vi "laser_LED_controls.vi"(1 "Pulse Duty Cycle":dbl=50.0 caption="%" min=0.0 max=100.0 step=0.1, 2 "Pulse 488":bool, 3 "Zelux Frequency":u16=10 caption="Hz", 11 "Running":bool) -> ()   [LabVIEW 2025]
uses:
  channel parameters cluster.ctl
  <vilib>/Utility/error.llb/DialogType.ctl
  <vilib>/DAQmx/write.llb/DAQmx Write (Analog 1D DBL NChan 1Samp).vi
  <vilib>/DAQmx/miscellaneous.llb/DAQmx Fill In Error Info.vi
panel:
  in  "488 nm LED control":dbl(slide) step=1.0 scale=0.0..100.0 scale format="%#_3g"
  out "488  nm voltage":dbl
  out "594 nm voltage":dbl
  in  "594 nm laser control":dbl(slide) step=1.0 scale=0.0..100.0 scale format="%#_3g"
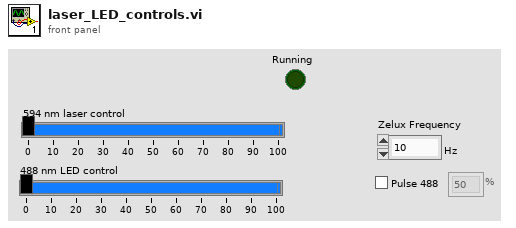
[diagram p1: front panel]
types:
  T1 = typedef "channel parameters cluster.ctl" = cluster{"voltage":dbl, "frequency":dbl, "duty cycle":dbl, "sample rate":dbl}
  T2 = typedef "DialogType.ctl" = u16
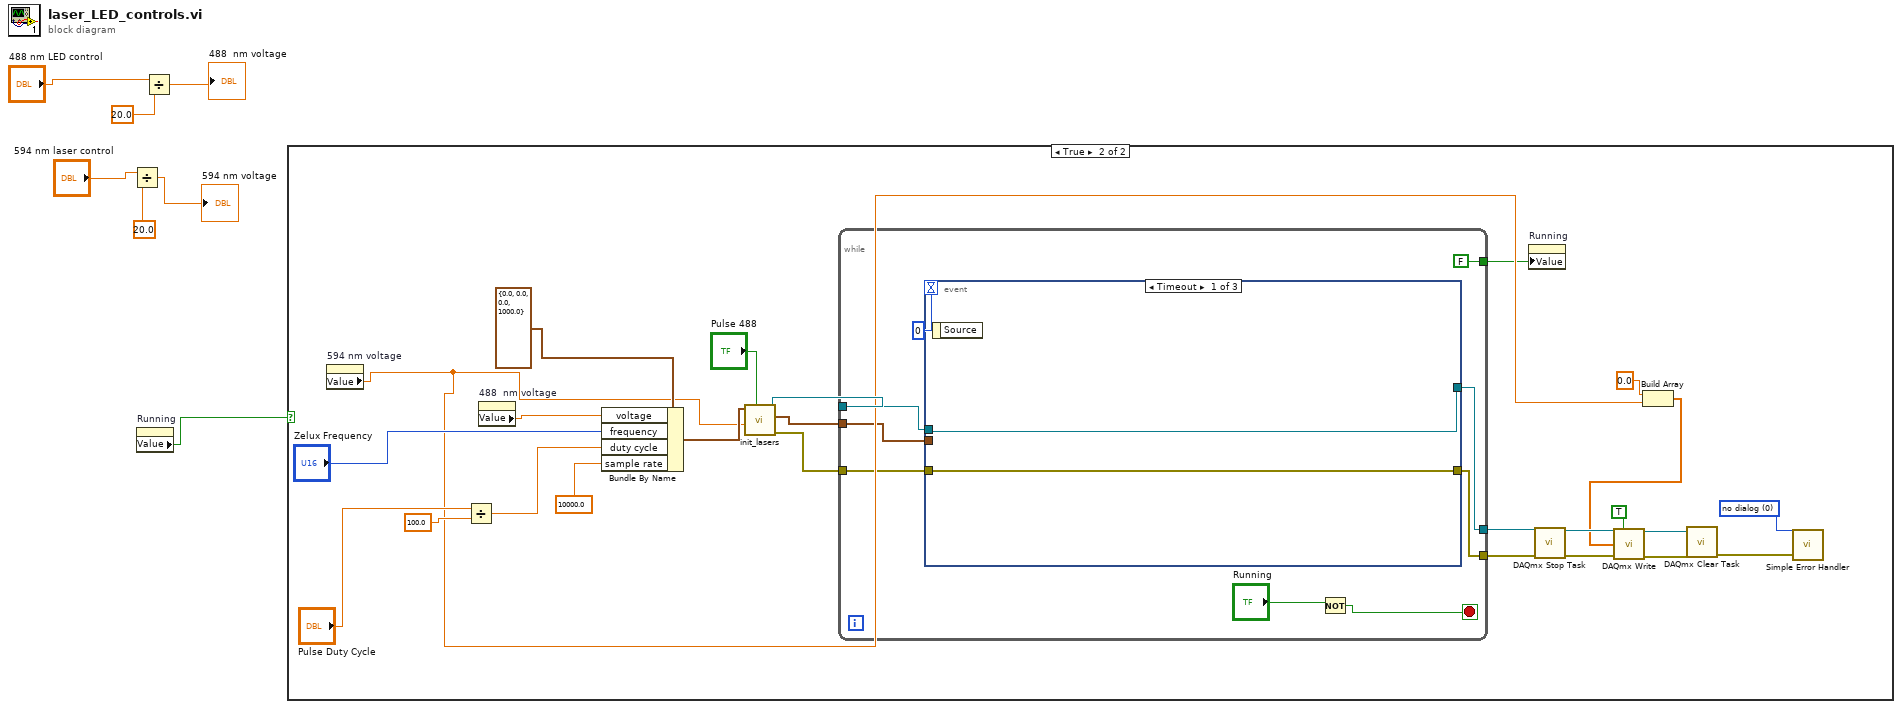
[diagram p0: block diagram]
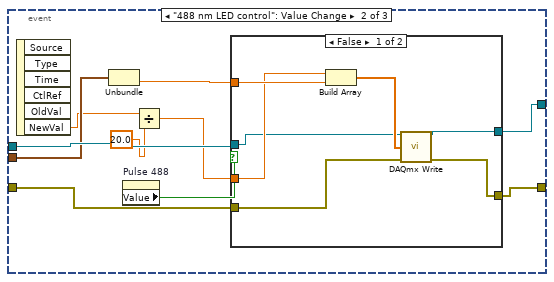
[diagram p3: hidden frame]
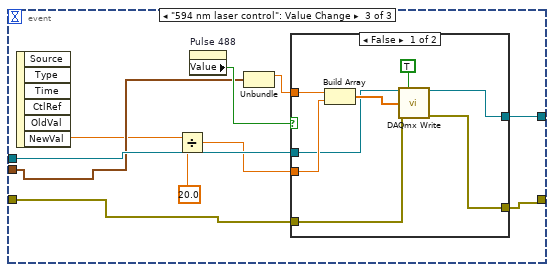
[diagram p5: hidden frame]
diagram:
  n1 = Divide(x="594 nm laser control", y=20.0) -> (x/y=→"594 nm voltage":dbl)
  n2 = property on="Running" class="Bool (strict)"() -> ("Value"=w1:bool)  [unwired: 2 in, 2 out]
  n3 = Divide(x="488 nm LED control", y=20.0) -> (x/y=→"488  nm voltage":dbl)
  n4 = case shown="True" w1 {
    frame False {
    }
    frame True {
      w22 = T2 0 items=["no dialog", "OK message", "continue or stop message", "OK message + warnings", "continue/stop + warnings"] ("type of dialog (OK msg:1)")
      n5 = property on="594 nm voltage" class="DigNum (strict)"() -> ("Value"=w13:dbl)  [unwired: 2 in, 2 out]
      n6 = Divide(x="Pulse Duty Cycle", y=100.0) -> (x/y=w30:dbl)
      n7 = property on="488  nm voltage" class="DigNum (strict)"() -> ("Value"=w27:dbl)  [unwired: 2 in, 2 out]
      n8 = Bundle By Name(cluster=T1 {"voltage"=0.0, "frequency"=0.0, "duty cycle"=0.0, "sample rate"=1000.0} ("channel parameters"), "voltage"=w27, "frequency"="Zelux Frequency", "duty cycle"=w30, "sample rate"=10000.0) -> (w32:T1)
      n9 = call "init_lasers.vi"("488 pulsed"="Pulse 488", "594 nm voltage"=w13, "488 nm channel parameters"=w32) -> ("error out"=w10:errorcluster, "current data"=w9:cluster{"[0]":dbl, "[1]":dbl}, "task out"=w15:refnum<k21>)  [unwired: 6 in]
      n10 = while {
        tunnel: w15 -> [w40]
        tunnel: w10 -> [w39]
        tunnel: [w38] -> w12
        tunnel: [w37] -> w11
        tunnel: w9 -> [w36]
        tunnel: [FALSE] -> w8
        stop <- w33 stop-if-true
        n11 = event shown="[0] Timeout" {
          selector: _ -> [_ _ _]
          dyn-events: _ -> [_ _ _]
          timeout: 0 -> [_ _ _]
          tunnel: w40 -> [w43 w51 w69]
          tunnel: w39 -> [w42 w52 w68]
          tunnel: [w43 w50 w70] -> w37
          tunnel: [w42 w47 w67] -> w38
          tunnel: w36 -> [_ w48 w66]
          event Timeout {
            n12 = event-data() -> ()  [unwired: 1 in, 1 out]
          }
          event "488 nm LED control": Value Change {
            n13 = event-data() -> ("NewVal"=w45:dbl)  [unwired: 1 in, 5 out]
            n14 = Unbundle(w48) -> ("[1]"=w49:dbl)  [unwired: 1 out]
            n15 = property on="Pulse 488" class="Bool (strict)"() -> ("Value"=w53:bool)  [unwired: 2 in, 2 out]
            n16 = Divide(x=w45, y=20.0) -> (x/y=w44:dbl)
            n17 = case shown="False" w53 {
              tunnel: [w59 w62] -> w47
              tunnel: w52 -> [w58 w62]
              tunnel: w51 -> [w54 w61]
              tunnel: [w57 w61] -> w50
              tunnel: w49 -> [w56 _]
              tunnel: w44 -> [w55 _]
              frame False {
                n18 = Build Array(w55, w56) -> (w60:dbl[])
                n19 = call-poly <vilib>:"DAQmx Write.vi"("task/channels in"=w54, "data"=w60, "error in"=w58) -> ("task out"=w57:refnum<k21>, "error out"=w59:errorcluster)  [unwired: 10 in, 1 out]
              }
              frame True {
              }
            }
          }
          event "594 nm laser control": Value Change {
            n20 = event-data() -> ("NewVal"=w64:dbl)  [unwired: 1 in, 5 out]
            n21 = Divide(x=w64, y=20.0) -> (x/y=w63:dbl)
            n22 = property on="Pulse 488" class="Bool (strict)"() -> ("Value"=w72:bool)  [unwired: 2 in, 2 out]
            n23 = Unbundle(w66) -> ("[0]"=w71:dbl)  [unwired: 1 out]
            n24 = case shown="False" w72 {
              tunnel: w71 -> [w80 _]
              tunnel: w63 -> [w79 _]
              tunnel: [w77 w82] -> w70
              tunnel: w69 -> [w76 w82]
              tunnel: w68 -> [w75 w81]
              tunnel: [w74 w81] -> w67
              frame False {
                n25 = Build Array(w80, w79) -> (w78:dbl[])
                n26 = call-poly <vilib>:"DAQmx Write.vi"("task/channels in"=w76, "auto start"=TRUE, "data"=w78, "error in"=w75) -> ("task out"=w77:refnum<k21>, "error out"=w74:errorcluster)  [unwired: 9 in, 1 out]
              }
              frame True {
              }
            }
          }
        }
        n27 = Not(x="Running") -> (.not. x?=w33:bool)
      }
      n28 = property on="Running" class="Bool (strict)"("Value"=w8) -> ()  [unwired: 2 in, 2 out]
      n29 = call <vilib>:"DAQmx Stop Task.vi"("task/channels in"=w11, "error in"=w12) -> ("task out"=w23:refnum<k21>, "error out"=w24:errorcluster)  [unwired: 12 in]
      n30 = Build Array(0.0 ("element"), w13) -> (w16:dbl[])
      n31 = call-poly <vilib>:"DAQmx Write.vi"("task/channels in"=w23, "auto start"=TRUE, "data"=w16, "error in"=w24) -> ("task out"=w20:refnum<k21>, "error out"=w19:errorcluster)  [unwired: 9 in, 1 out]
      n32 = call <vilib>:"DAQmx Clear Task.vi"("task in"=w20, "error in"=w19) -> ("error out"=w21:errorcluster)  [unwired: 13 in]
      n33 = call <vilib>:"Simple Error Handler.vi"("type of dialog (OK msg:1)"=w22, "error in (no error)"=w21) -> ()  [unwired: 3 in, 5 out]
    }
  }
